vi "Read UI Constans.vi"(8 "error in (no error)":errorcluster, 11 "CFG File Refnum in":T2) -> (0 "error out":errorcluster, 2 "Controller 2":T1, 3 "CFG File Refnum out":T2)   [LabVIEW 2017]
uses:
  <vilib>/Utility/config.llb/Config Data RefNum.ctl
  Car Wash System Globals.vi
  <vilib>/Utility/config.llb/Read Key (Double).vi
  <vilib>/Utility/error.llb/Error Cluster From Error Code.vi
  <vilib>/ErrorRing/Error Ring.xnode
  <vilib>/Utility/config.llb/NI_LVConfig.lvlib
panel:
  in  "Controller":T1
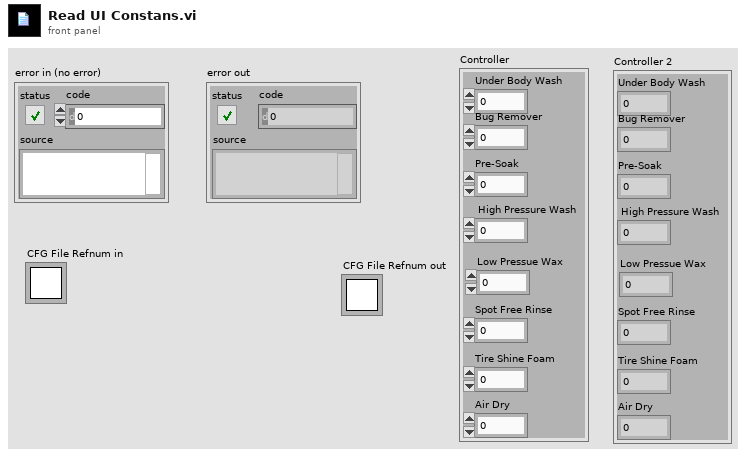
[diagram p1: front panel]
types:
  T1 = typedef "Configuration Data — Controller.ctl" = cluster{"Under Body Wash ":dbl, "Bug Remover":dbl, "Pre-Soak":dbl, " High Pressure Wash":dbl, "Low Pressue Wax ":dbl, "Spot Free Rinse ":dbl, "Tire Shine Foam":dbl, "Air Dry ":dbl}
  T2 = typedef "NI_LVConfig.lvlib/Config Data RefNum.ctl" = refnum<k1>
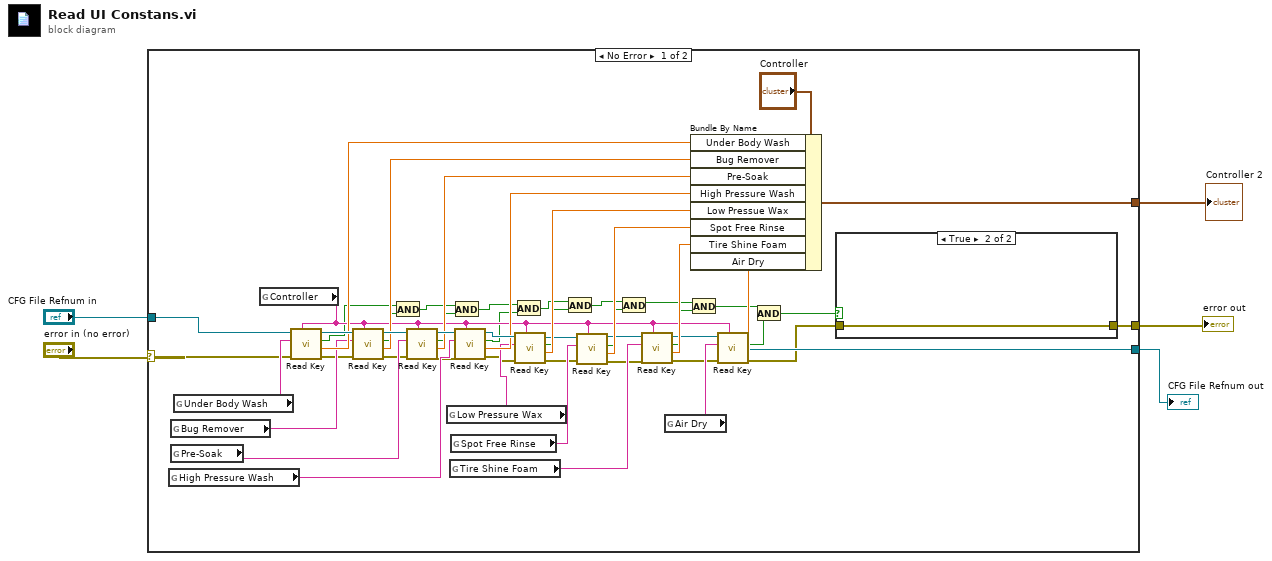
[diagram p0: block diagram]
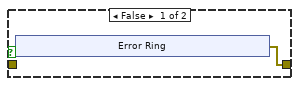
[diagram p2: hidden frame]
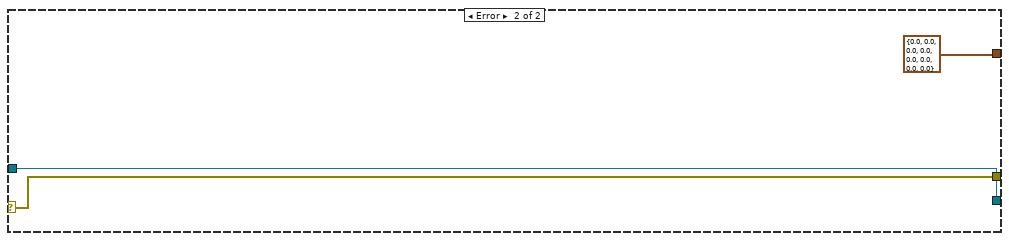
[diagram p3: hidden frame]
diagram:
  n1 = case shown="No Error" "error in (no error)" {
    selector: "error in (no error)" -> [w33 w68]
    tunnel: [w7 w68] -> w4
    tunnel: "CFG File Refnum in" -> [w58 w67]
    tunnel: [w45 T1 {"Under Body Wash "=0.0, "Bug Remover"=0.0, "Pre-Soak"=0.0, " High Pressure Wash"=0.0, "Low Pressue Wax "=0.0, "Spot Free Rinse "=0.0, "Tire Shine Foam"=0.0, "Air Dry "=0.0} ("Controller")] -> w1
    tunnel: [w24 w67] -> w2
    frame No Error {
      n2 = global read "Car Wash System Globals.vi" "High Pressure Wash"() -> (w44:string)
      n3 = global read "Car Wash System Globals.vi" "Bug Remover"() -> (w47:string)
      n4 = global read "Car Wash System Globals.vi" "Pre-Soak"() -> (w46:string)
      n5 = global read "Car Wash System Globals.vi" "Under Body Wash"() -> (w53:string)
      n6 = global read "Car Wash System Globals.vi" "Controller"() -> (w25:string)
      n7 = call-poly <vilib>:"Read Key.vi"("section"=w25, "error in (no error)"=w33, "key"=w53, "refnum"=w58) -> ("error out"=w32:errorcluster, "value"=w52:dbl, "found?"=w23:bool, "refnum out"=w57:T2)  [unwired: 4 in]
      n8 = call-poly <vilib>:"Read Key.vi"("section"=w25, "error in (no error)"=w32, "key"=w47, "refnum"=w57) -> ("error out"=w31:errorcluster, "value"=w51:dbl, "found?"=w22:bool, "refnum out"=w56:T2)  [unwired: 4 in]
      n9 = And(x=w23, y=w22) -> (x .and. y?=w21:bool)
      n10 = call-poly <vilib>:"Read Key.vi"("section"=w25, "error in (no error)"=w31, "key"=w46, "refnum"=w56) -> ("error out"=w30:errorcluster, "value"=w50:dbl, "found?"=w20:bool, "refnum out"=w55:T2)  [unwired: 4 in]
      n11 = global read "Car Wash System Globals.vi" "Low Pressure Wax"() -> (w40:string)
      n12 = global read "Car Wash System Globals.vi" "Tire Shine Foam"() -> (w38:string)
      n13 = global read "Car Wash System Globals.vi" "Spot Free Rinse"() -> (w39:string)
      n14 = And(x=w21, y=w20) -> (x .and. y?=w18:bool)
      n15 = call-poly <vilib>:"Read Key.vi"("section"=w25, "error in (no error)"=w30, "key"=w44, "refnum"=w55) -> ("error out"=w29:errorcluster, "value"=w49:dbl, "found?"=w19:bool, "refnum out"=w54:T2)  [unwired: 4 in]
      n16 = And(x=w18, y=w19) -> (x .and. y?=w16:bool)
      n17 = call-poly <vilib>:"Read Key.vi"("section"=w25, "error in (no error)"=w29, "key"=w40, "refnum"=w54) -> ("error out"=w28:errorcluster, "value"=w48:dbl, "found?"=w17:bool, "refnum out"=w34:T2)  [unwired: 4 in]
      n18 = And(x=w16, y=w17) -> (x .and. y?=w14:bool)
      n19 = call-poly <vilib>:"Read Key.vi"("section"=w25, "error in (no error)"=w28, "key"=w39, "refnum"=w34) -> ("error out"=w27:errorcluster, "value"=w43:dbl, "found?"=w15:bool, "refnum out"=w35:T2)  [unwired: 4 in]
      n20 = And(x=w14, y=w15) -> (x .and. y?=w12:bool)
      n21 = call-poly <vilib>:"Read Key.vi"("section"=w25, "error in (no error)"=w27, "key"=w38, "refnum"=w35) -> ("error out"=w26:errorcluster, "value"=w42:dbl, "found?"=w13:bool, "refnum out"=w36:T2)  [unwired: 4 in]
      n22 = global read "Car Wash System Globals.vi" "Air Dry"() -> (w37:string)
      n23 = And(x=w12, y=w13) -> (x .and. y?=w10:bool)
      n24 = call-poly <vilib>:"Read Key.vi"("section"=w25, "error in (no error)"=w26, "key"=w37, "refnum"=w36) -> ("error out"=w8:errorcluster, "value"=w41:dbl, "found?"=w11:bool, "refnum out"=w24:T2)  [unwired: 4 in]
      n25 = Bundle By Name(cluster="Controller", "Under Body Wash"=w52, "Bug Remover"=w51, "Pre-Soak"=w50, "High Pressure Wash"=w49, "Low Pressue Wax"=w48, "Spot Free Rinse"=w43, "Tire Shine Foam"=w42, "Air Dry"=w41) -> (w45:T1)
      n26 = And(x=w10, y=w11) -> (x .and. y?=w9:bool)
      n27 = case shown="True" w9 {
        tunnel: w8 -> [_ w65]
        tunnel: [w59 w65] -> w7
        frame False {
          n28 = xnode "Error Ring"() -> ("error out"=w59:errorcluster)
        }
        frame True {
        }
      }
    }
    frame Error {
    }
  }
  "error out" <- w4
  "CFG File Refnum out" <- w2
  "Controller 2" <- w1
